vi "Set Gain1.vi"(0 "NMR in":refnum<class "NMR.lvclass">, 5 "Gain (dB)":i8=15 min=-5 max=45 step=1, 11 "error in (no error)":errorcluster) -> (4 "NMR out":refnum<class "NMR.lvclass">, 10 "String as ASCII":string, 15 "error out":errorcluster)   [LabVIEW 2011, in "NMR.lvclass"]
uses:
  NMR.lvclass
panel:
  in  "Numeric 2":fxp<+,12,12>
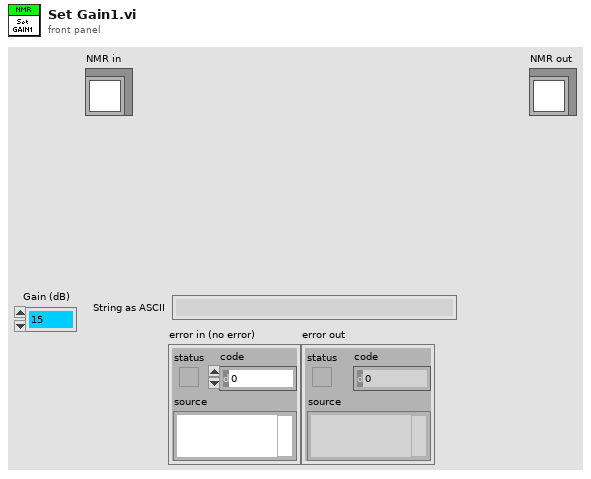
[diagram p1: front panel]
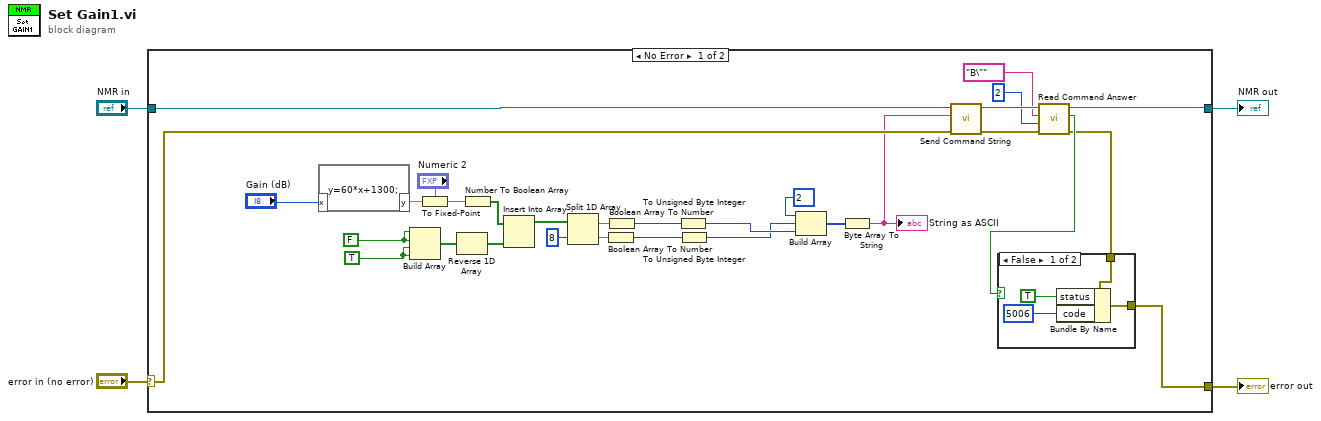
[diagram p0: block diagram]
diagram:
  n1 = case shown="No Error" "error in (no error)" {
    selector: "error in (no error)" -> [w31 w41]
    tunnel: [w22 w41] -> w3
    tunnel: [w32 w40] -> w1
    tunnel: "NMR in" -> [w34 w40]
    frame No Error {
      w19 = TRUE ("element")
      w7 = FALSE ("A/B")
      n2 = formula code="y=60*x+1300;"("x"="Gain (dB)") -> ("y"=w16:dbl)
      n3 = Build Array(w7, w7, w19, w19) -> (w20:bool[])
      n4 = To Fixed-Point(fixed-point type="Numeric 2", number=w16) -> (fixed-point=w15:fxp<+,12,12>)
      n5 = Reverse 1D Array(array=w20) -> (reversed array=w18:bool[])
      n6 = Number To Boolean Array(number=w15) -> (Boolean array=w14:bool[])
      n7 = Insert Into Array(array=w14, new element=w18) -> (w10:bool[])  [unwired: 1 in]
      n8 = Split 1D Array(array=w10, index=8) -> (first subarray=w12:bool[], second subarray=w11:bool[])
      n9 = Boolean Array To Number(Boolean array=w11) -> (number=w8:u32)
      n10 = Boolean Array To Number(Boolean array=w12) -> (number=w9:u32)
      n11 = To Unsigned Byte Integer(number=w9) -> (unsigned 8bit integer=w6:u8)
      n12 = To Unsigned Byte Integer(number=w8) -> (unsigned 8bit integer=w5:u8)
      n13 = Build Array(u32 2 ("element"), w5, w6) -> (w29:u32[])
      n14 = Byte Array To String(unsigned byte array=w29) -> (string=w27:string)
      "String as ASCII" <- w27
      n15 = call-dynamic "Send Command String.vi"("error in (no error)"=w31, "Command String"=w27, "NMR in"=w34) -> ("error out"=w30:errorcluster, "NMR out"=w33:refnum<class "NMR.lvclass">)  [unwired: 7 in]
      n16 = call-dynamic "Read Command Answer.vi"("error in (no error)"=w30, "bytes to read"=u32 2 ("Number bytes Read"), "String Seached"="B\"" ("search char"), "NMR in"=w33) -> ("error out"=w23:errorcluster, "Expected Answer?"=w24:bool, "NMR out"=w32:refnum<class "NMR.lvclass">)  [unwired: 5 in]
      n17 = case shown="False" w24 {
        tunnel: w23 -> [w36 w39]
        tunnel: [w35 w39] -> w22
        frame False {
          n18 = Bundle By Name(cluster=w36, "status"=TRUE, "code"=5006) -> (w35:errorcluster)
        }
        frame True {
        }
      }
    }
    frame Error {
    }
  }
  "error out" <- w3
  "NMR out" <- w1
